vi "scale xy steering.vi"(8 "0 to 9 V input":dbl, 11 "-2.5 to 2.5 V input":dbl) -> (0 "-2.5 to 2.5 V output":dbl, 3 "0 to 9 V output":dbl)   [LabVIEW 2012]
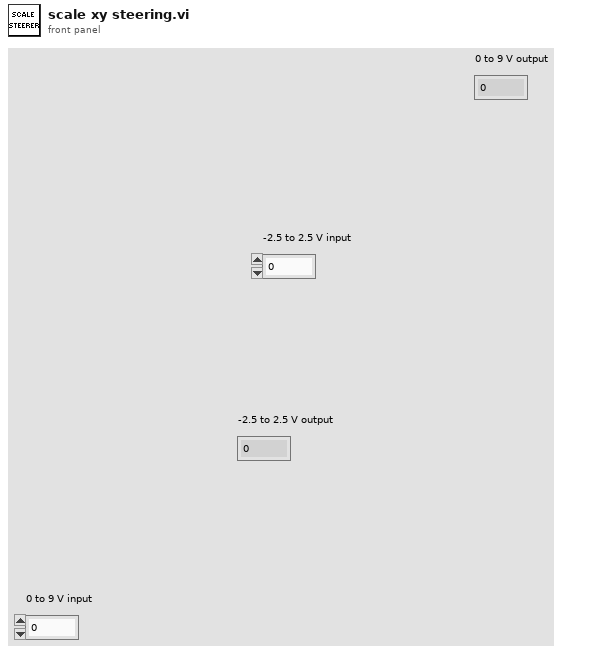
[diagram p1: front panel]
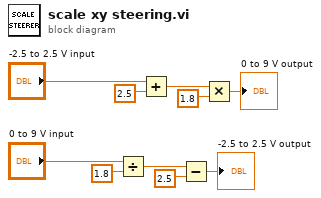
[diagram p0: block diagram]
diagram:
  n1 = Divide(x="0 to 9 V input", y=1.8) -> (x/y=w2:dbl)
  n2 = Add(x="-2.5 to 2.5 V input", y=2.5) -> (x+y=w8:dbl)
  n3 = Subtract(x=w2, y=2.5) -> (x-y=→"-2.5 to 2.5 V output":dbl)
  n4 = Multiply(x=w8, y=1.8) -> (x*y=→"0 to 9 V output":dbl)
